vi "Modbus Register Write.vi"(8 "error in":errorcluster, 11 "Alabama Power Remote in":refnum<class "Alabama Power Remote.lvclass">) -> (0 "error out":errorcluster, 3 "Alabama Power Remote out":refnum<class "Alabama Power Remote.lvclass">)   [LabVIEW 2018, in "Alabama Power Remote Actor.lvlib" / "Alabama Power Remote.lvclass"]
uses:
  Alabama Power Remote.lvclass
  C:/Users/Administrator/Desktop/2018LabVIEW EMS/Remote Operation/Remote Operation Abstract/Remote Operation Abstract.lvclass
  C:/Users/Administrator/Desktop/2018LabVIEW EMS/EMS Generic Actor/EMS Generic/EMS Generic.lvclass
  Alabama Power Remote.lvclass/Alabama Power Remote.ctl
  <vilib>/Modbus/master/Modbus Master.lvclass
  EMS Generic Actor/EMS Generic/EMS Generic.lvclass
  Remote Operation Abstract/Remote Operation Abstract.lvclass
panel:
  in  "Island Fail":bool
  in  "Resynchronize Fail":bool
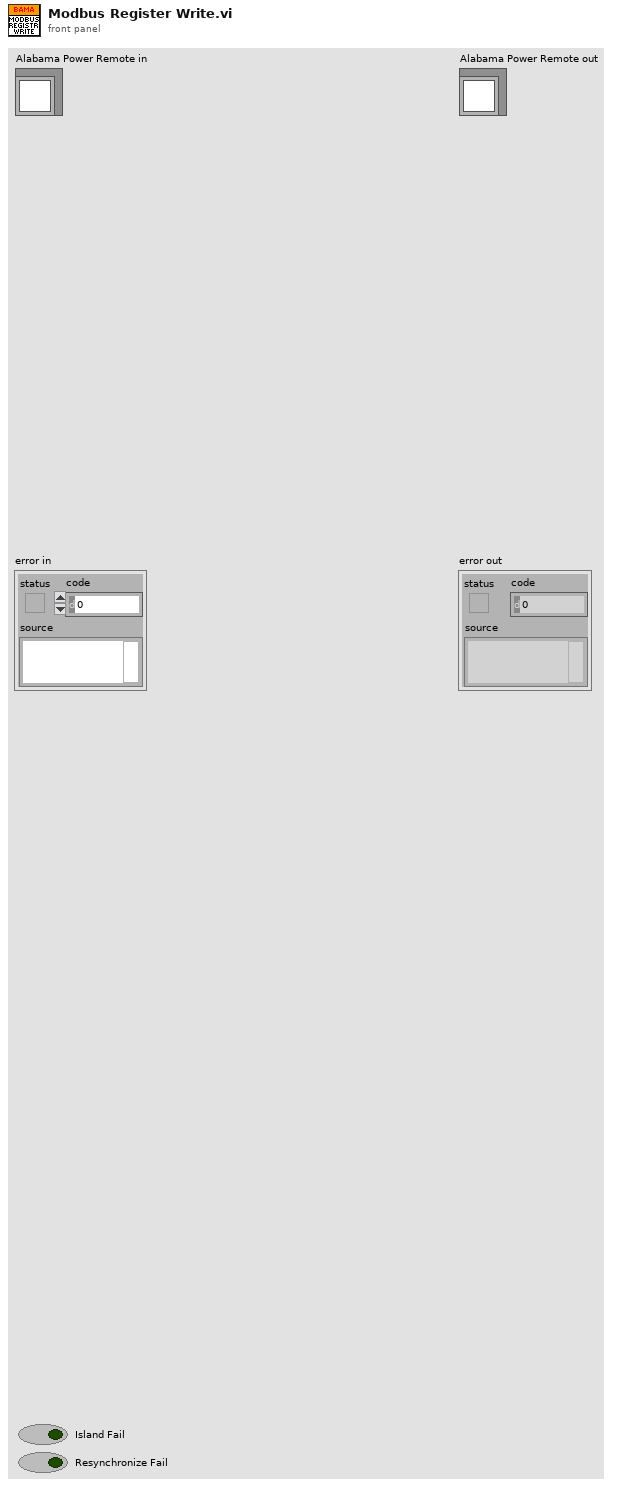
[diagram p1: front panel]
types:
  T1 = typedef "CSEISMIC DDS.lvlib/CSEISMIC DDS.lvclass/DeviceID.ctl" = string
  T2 = typedef "CSEISMIC DDS.lvlib/CSEISMIC DDS.lvclass/DER_Measurement.ctl" = cluster{"DeviceID":T1, "Voltage":dbl[], "Current":dbl[], "RealPower":dbl[], "ReactivePower":dbl[], "LineConfig":u8[], "Frequency":dbl}
  T3 = typedef "CSEISMIC DDS.lvlib/CSEISMIC DDS.lvclass/IED_Status.ctl" = cluster{"DeviceID":T1, "Timestamp":T4, "MicrogridID":u8, "Active":bool, "Inactive":bool, "Error":i32, "Fault":bool, "ErrorString":string}
  T4 = typedef "CSEISMIC DDS.lvlib/CSEISMIC DDS.lvclass/Timestamp.ctl" = cluster{"Seconds":u64, "Remainder":u64}
  T5 = typedef "CSEISMIC DDS.lvlib/CSEISMIC DDS.lvclass/SmartRelay_Measurement.ctl" = cluster{"DeviceID":T1, "PrimaryVoltage":dbl[], "SecondaryVoltage":dbl[], "Current":dbl[], "RealPower":dbl[], "ReactivePower":dbl[], "LineConfig":u8[], "Frequency":dbl}
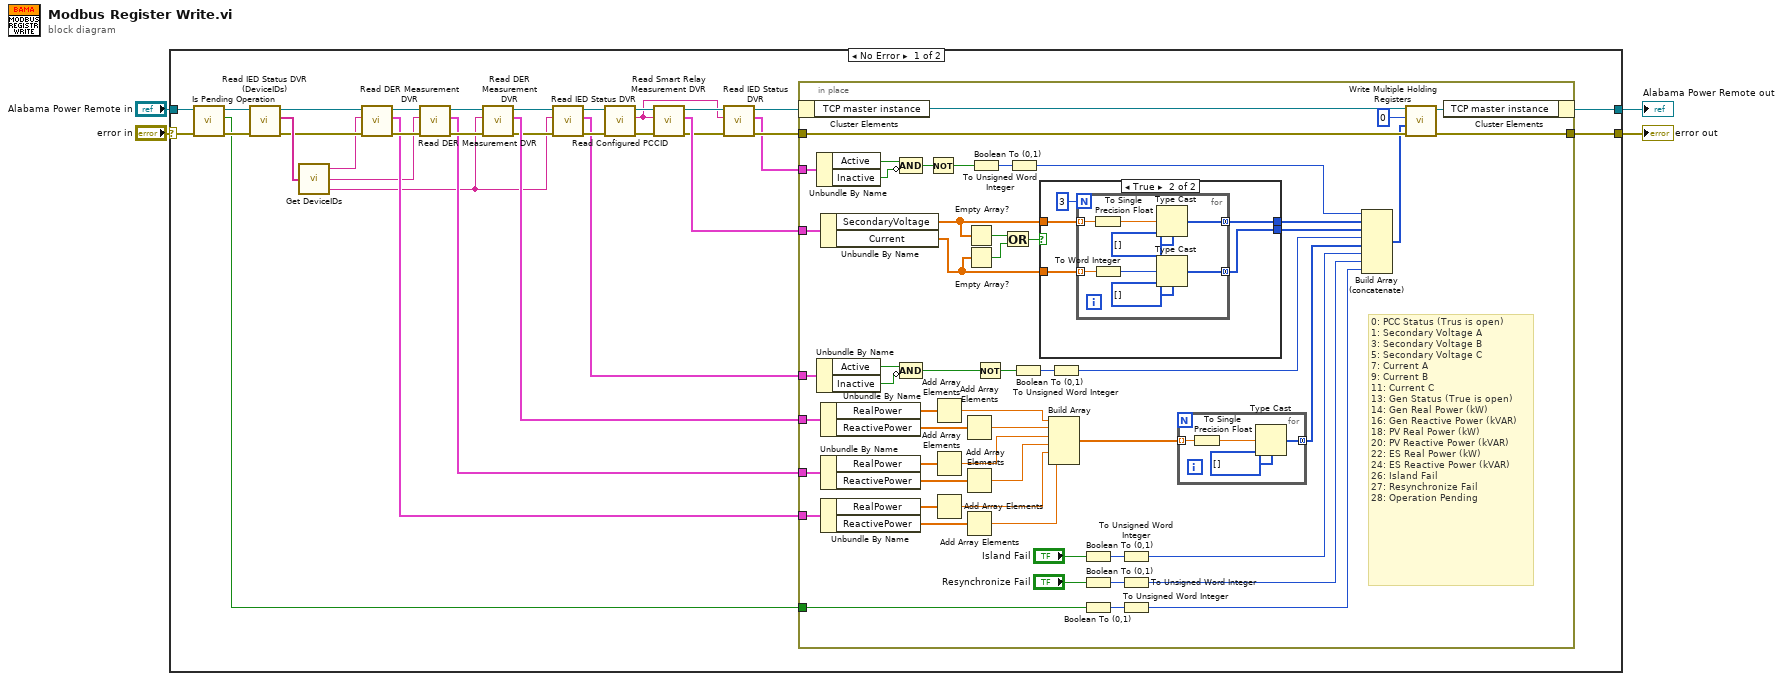
[diagram p0: block diagram]
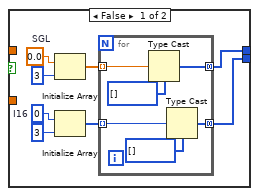
[diagram p2: hidden frame]
diagram:
  n1 = case shown="No Error" "error in" {
    selector: "error in" -> [w7 w125]
    tunnel: [w38 w125] -> w3
    tunnel: [w37 w124] -> w1
    tunnel: "Alabama Power Remote in" -> [w9 w124]
    frame No Error {
      n2 = call "Is Pending Operation.vi"("error in"=w7, "Remote Operation Abstract"=w9) -> ("error out"=w6:errorcluster, "Pending?"=w5:bool, "dup Remote Operation Abstract"=w8:refnum<class "Alabama Power Remote.lvclass">)  [unwired: 7 in]
      n3 = call "Read IED Status DVR (DeviceIDs).vi"("error in"=w6, "EMS Generic in"=w8) -> ("error out"=w22:errorcluster, "DeviceID Array"=w33:T1[], "EMS Generic out"=w25:refnum<class "Alabama Power Remote.lvclass">)  [unwired: 7 in]
      n4 = call "Get DeviceIDs.vi"("DeviceID Array"=w33) -> ("ES DeviceID"=w16:T1, "PV DeviceID"=w17:T1, "Gen DeviceID"=w11:T1)
      n5 = call "Read DER Measurement DVR.vi"("error in"=w22, "DeviceID"=w16, "EMS Generic in"=w25) -> ("error out"=w21:errorcluster, "DER_Measurement"=w18:T2, "EMS Generic out"=w24:refnum<class "Alabama Power Remote.lvclass">)  [unwired: 5 in, 1 out]
      n6 = call "Read DER Measurement DVR.vi"("error in"=w21, "DeviceID"=w17, "EMS Generic in"=w24) -> ("error out"=w20:errorcluster, "DER_Measurement"=w19:T2, "EMS Generic out"=w23:refnum<class "Alabama Power Remote.lvclass">)  [unwired: 5 in, 1 out]
      n7 = call "Read DER Measurement DVR.vi"("error in"=w20, "DeviceID"=w11, "EMS Generic in"=w23) -> ("error out"=w12:errorcluster, "DER_Measurement"=w32:T2, "EMS Generic out"=w15:refnum<class "Alabama Power Remote.lvclass">)  [unwired: 5 in, 1 out]
      n8 = call "Read IED Status DVR.vi"("error in"=w12, "DeviceID"=w11, "EMS Generic in"=w15) -> ("error out"=w13:errorcluster, "IED_Status"=w10:T3, "EMS Generic out"=w14:refnum<class "Alabama Power Remote.lvclass">)  [unwired: 5 in, 1 out]
      n9 = call "Read Configured PCCID.vi"("error in"=w13, "EMS Generic in"=w14) -> ("error out"=w36:errorcluster, "PCCID"=w27:T1, "EMS Generic out"=w35:refnum<class "Alabama Power Remote.lvclass">)  [unwired: 7 in]
      n10 = call "Read Smart Relay Measurement DVR.vi"("error in"=w36, "DeviceID"=w27, "EMS Generic in"=w35) -> ("error out"=w29:errorcluster, "SmartRelay_Measurement"=w34:T5, "EMS Generic out"=w31:refnum<class "Alabama Power Remote.lvclass">)  [unwired: 5 in, 1 out]
      n11 = call "Read IED Status DVR.vi"("error in"=w29, "DeviceID"=w27, "EMS Generic in"=w31) -> ("error out"=w28:errorcluster, "IED_Status"=w26:T3, "EMS Generic out"=w30:refnum<class "Alabama Power Remote.lvclass">)  [unwired: 5 in, 1 out]
      n12 = in-place {
        in-place-border: w28 -> [w90]
        in-place-border: [w89] -> w38
        in-place-border: w34 -> [w87]
        in-place-border: w32 -> [w84]
        in-place-border: w26 -> [w85]
        in-place-border: w19 -> [w72]
        in-place-border: w18 -> [w73]
        in-place-border: w10 -> [w83]
        in-place-border: w5 -> [w50]
        # "0: PCC Status (Trus is open)\n1: Secondary Voltage A\n3: Secondary Voltage B\n5: Secondary Voltage C\n7: Current A\n9: Current B\n11: Current C\n13: Gen Status (True is open)\n14: Gen Real Power (kW)\n16: Gen Reactive Power (kVAR)\n18: PV Real Power (kW)\n20: PV Reactive Power (kVAR)\n22: ES Real Power (kW)\n24: ES Reactive Power (kVAR)\n26: Island Fail\n27: Resynchronize Fail\n28: Operation Pending"
        n13 = in-place-cluster #1(w30) -> ("TCP master instance"=w92:refnum<class "Modbus Master.lvclass">)
        n14 = Unbundle By Name(w85) -> ("Active"=w46:bool, "Inactive"=w45:bool)
        n15 = Unbundle By Name(w83) -> ("Active"=w49:bool, "Inactive"=w48:bool)
        n16 = Unbundle By Name(w87) -> ("SecondaryVoltage"=w43:dbl[], "Current"=w42:dbl[])
        n17 = Unbundle By Name(w84) -> ("RealPower"=w81:dbl[], "ReactivePower"=w80:dbl[])
        n18 = Unbundle By Name(w72) -> ("RealPower"=w76:dbl[], "ReactivePower"=w77:dbl[])
        n19 = Unbundle By Name(w73) -> ("RealPower"=w75:dbl[], "ReactivePower"=w74:dbl[])
        n20 = Compound Arithmetic op=AND(w46, invert w45) -> (w44:bool)
        n21 = Compound Arithmetic op=AND(w49, invert w48) -> (w47:bool)
        n22 = Not(x=w44) -> (.not. x?=w51:bool)
        n23 = Add Array Elements(numeric array=w81) -> (sum=w79:dbl)
        n24 = Add Array Elements(numeric array=w76) -> (sum=w71:dbl)
        n25 = Add Array Elements(numeric array=w75) -> (sum=w69:dbl)
        n26 = Add Array Elements(numeric array=w80) -> (sum=w78:dbl)
        n27 = Add Array Elements(numeric array=w77) -> (sum=w70:dbl)
        n28 = Add Array Elements(numeric array=w74) -> (sum=w68:dbl)
        n29 = Empty Array?(array=w43) -> (empty?=w41:bool)
        n30 = Empty Array?(array=w42) -> (empty?=w40:bool)
        n31 = Boolean To (0,1)(Boolean=w51) -> (0, 1=w66:i16)
        n32 = Not(x=w47) -> (.not. x?=w52:bool)
        n33 = Or(x=w41, y=w40) -> (x .or. y?=w39:bool)
        n34 = To Unsigned Word Integer(number=w66) -> (unsigned 16bit integer=w65:u16)
        n35 = Boolean To (0,1)(Boolean=w52) -> (0, 1=w64:i16)
        n36 = case shown="True" w39 {
          tunnel: [w97 w111] -> w82
          tunnel: [w93 w109] -> w54
          tunnel: w43 -> [_ w108]
          tunnel: w42 -> [_ w107]
          frame False {
            w96 = i16 0  # I16
            w99 = sgl 0.0  # SGL
            n37 = Initialize Array(w99, 3 ("dimension size")) -> (w98:sgl[])
            n38 = Initialize Array(w96, 3 ("dimension size")) -> (w94:i16[])
            n39 = for {
              tunnel: w98 -> [w105] mode=indexing
              tunnel: [w103] -> w97 mode=concatenating
              tunnel: w94 -> [w102] mode=indexing
              tunnel: [w101] -> w93 mode=concatenating
              n40 = Type Cast(type=u16[] [] ("16bit integer"), x=w105) -> (*(type *) &x=w103:u16[])
              n41 = Type Cast(type=u16[] [] ("16bit integer"), x=w102) -> (*(type *) &x=w101:u16[])
            }
          }
          frame True {
            n42 = for {
              N: 3 -> [_]
              tunnel: w108 -> [w119] mode=indexing
              tunnel: [w117] -> w111 mode=concatenating
              tunnel: [w113] -> w109 mode=concatenating
              tunnel: w107 -> [w112] mode=indexing
              n43 = To Single Precision Float(number=w119) -> (single precision float=w118:sgl)
              n44 = To Word Integer(number=w112) -> (16bit integer=w114:i16)
              n45 = Type Cast(type=u16[] [] ("16bit integer"), x=w118) -> (*(type *) &x=w117:u16[])
              n46 = Type Cast(type=u16[] [] ("16bit integer"), x=w114) -> (*(type *) &x=w113:u16[])
            }
          }
        }
        n47 = Build Array(w79, w78, w71, w70, w69, w68) -> (w53:dbl[])
        n48 = To Unsigned Word Integer(number=w64) -> (unsigned 16bit integer=w63:u16)
        n49 = Boolean To (0,1)(Boolean="Island Fail") -> (0, 1=w58:i16)
        n50 = Boolean To (0,1)(Boolean="Resynchronize Fail") -> (0, 1=w61:i16)
        n51 = Boolean To (0,1)(Boolean=w50) -> (0, 1=w62:i16)
        n52 = To Unsigned Word Integer(number=w58) -> (unsigned 16bit integer=w57:u16)
        n53 = To Unsigned Word Integer(number=w61) -> (unsigned 16bit integer=w56:u16)
        n54 = To Unsigned Word Integer(number=w62) -> (unsigned 16bit integer=w55:u16)
        n55 = for {
          tunnel: w53 -> [w123] mode=indexing
          tunnel: [w121] -> w67 mode=concatenating
          n56 = To Single Precision Float(number=w123) -> (single precision float=w122:sgl)
          n57 = Type Cast(type=u16[] [] ("16bit integer"), x=w122) -> (*(type *) &x=w121:u16[])
        }
        n58 = Build Array (concatenate)(w65, w82, w54, w63, w67, w57, w56, w55) -> (w86:u16[])
        n59 = call-dynamic "Write Multiple Holding Registers.vi"("error in (no error)"=w90, "holding register values"=w86, "starting address"=u16 0, "Modbus master in"=w92) -> ("error out"=w89:errorcluster, "Modbus master out"=w91:refnum<class "Modbus Master.lvclass">)  [unwired: 6 in]
        n60 = in-place-cluster #1("TCP master instance"=w91) -> (w37:refnum<class "Alabama Power Remote.lvclass">)
      }
    }
    frame Error {
    }
  }
  "error out" <- w3
  "Alabama Power Remote out" <- w1
